vi "WirebondPatMatch.vi"(6 "Minimum Match Score":sgl, 7 "controller in":refnum<k24>, 8 "Template":path, 9 "Top or Bottom":dbl) -> (0 "error out":errorcluster, 1 "Number of Matches":i32, 3 "Match(es) Found":bool)   [LabVIEW 2011]
uses:
  <vilib>/vision/Pattern Matching.llb/IMAQ GM Match Report.ctl
  C:/Users/Admin/Desktop/Gantry Code Transfer/source/Code Transfer/Aerotech.A3200.dll
  Aerotech.A3200.dll
  Template change for pattern match.vi
  <vilib>/vision/driver/NI_Vision_Acquisition_Software.lvlib
  <vilib>/vision/NI_Vision_Development_Module.lvlib
  C:/Program Files/National Instruments/LabVIEW 2011/resource/objmgr/imaqdx.rc
panel:
  in  "Max":dbl=60.0
  in  "Min":dbl
  in  "Scale Factor":sgl=0.000429
  out "y rel move":dbl
  out "x rel move":dbl
  out "y":sgl
  out "x":sgl
  out "Image Out":T1(plugin-control)
  out "Calibrated Matches":T2[](array[typedef]) {"Correlation Score" format="%.2f"; "Target Template Curve Score" format="%.2f"; "Template Target Curve Score" format="%.2f"; "Bounding Box"."y" format="%.2f"; "Bounding Box"."x" format="%.2f"; "Position"."y" format="%.2f"; "Position"."x" format="%.2f"; "Score" format="%.2f"; "Scale" format="%.2f"; "Angle" format="%.2f"; "Occlusion %" format="%.2f"}
  out "Matches":T2[](array[typedef]) {"Correlation Score" format="%.2f"; "Target Template Curve Score" format="%.2f"; "Template Target Curve Score" format="%.2f"; "Bounding Box"."y" format="%.2f"; "Bounding Box"."x" format="%.2f"; "Position"."y" format="%.2f"; "Position"."x" format="%.2f"; "Score" format="%.2f"; "Scale" format="%.2f"; "Angle" format="%.2f"; "Occlusion %" format="%.2f"}
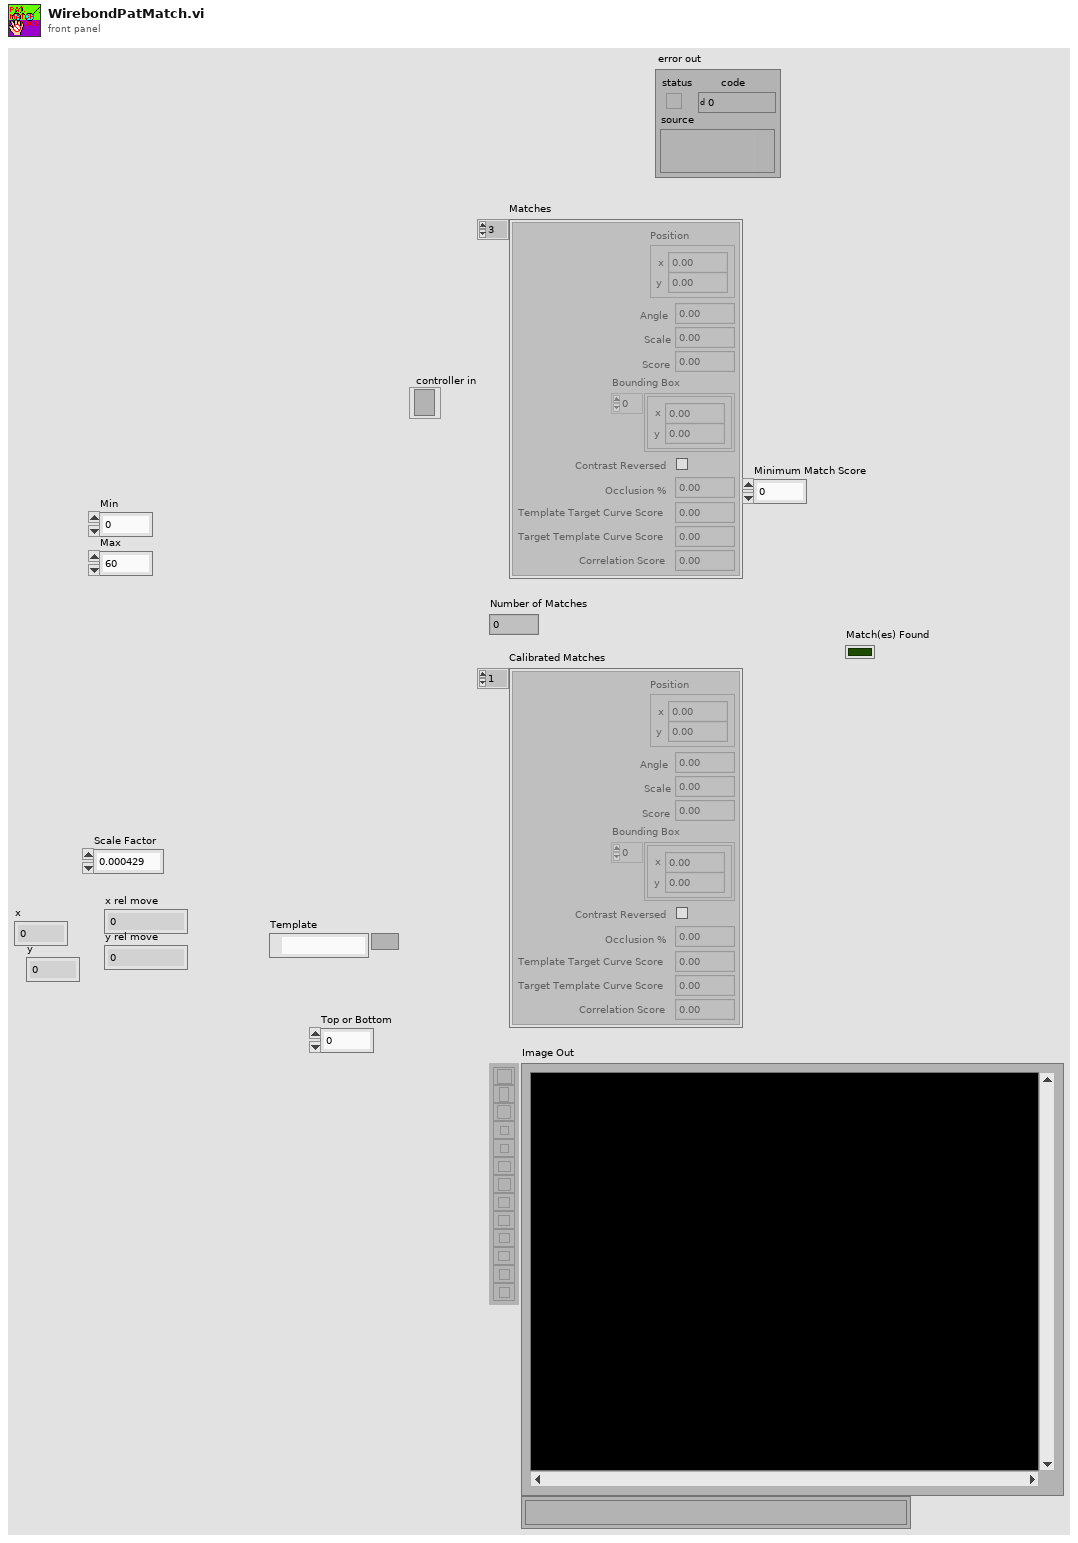
[diagram p1: front panel]
types:
  T1 = typedef "IMAQ Image.ctl" = refnum<image>
  T2 = typedef "IMAQ GM Match Report.ctl" = cluster{"Position":cluster{"x":sgl, "y":sgl}, "Angle":sgl, "Scale":sgl, "Score":sgl, "Bounding Box":cluster{"x":sgl, "y":sgl}[], "Contrast Reversed":bool, "Occlusion %":sgl, "Template Target Curve Score":sgl, "Target Template Curve Score":sgl, "Correlation Score":sgl}
  T3 = cluster{"Curve Parameters":cluster{"Extraction Mode":u32, "Edge Threshold":i32, "Edge Filter Size":u32, "Min Length":i32, "Row Search Step Size":i32, "Col Search Step Size":i32, "Max Endpoint Gap":i32, "Closed":bool, "Subpixel":bool}, "Match Mode":cluster{"Rotation":bool, "Scale":bool, "Occlusion":bool, "Reserved":bool, "Reserved":bool, "Reserved":bool}, "Range Settings":cluster{"Match Constraints":u32, "Min":dbl, "Max":dbl}[], "Number of Matches Requested":i32, "Minimum Match Score":sgl, "Subpixel Accuracy":bool}
  T4 = cluster{"Global Rectangle":i32[], "Contours":cluster{"ID":enum32{"External", "Internal"}, "Type":u32, "Coordinates":i32[]}[]}
  T5 = typedef "IMAQdx.ctl" = refnum<k21>
  T6 = cluster{"Extraction Mode":u32, "Edge Threshold":i32, "Edge Filter Size":u32, "Min Length":i32, "Row Search Step Size":i32, "Col Search Step Size":i32, "Max Endpoint Gap":i32, "Closed":bool, "Subpixel":bool}
  T7 = cluster{"Rotation":bool, "Scale":bool, "Occlusion":bool, "Reserved":bool, "Reserved":bool, "Reserved":bool}
  T8 = cluster{"Match Constraints":u32, "Min":dbl, "Max":dbl}[]
  T9 = cluster{"Match Constraints":u32, "Min":dbl, "Max":dbl}
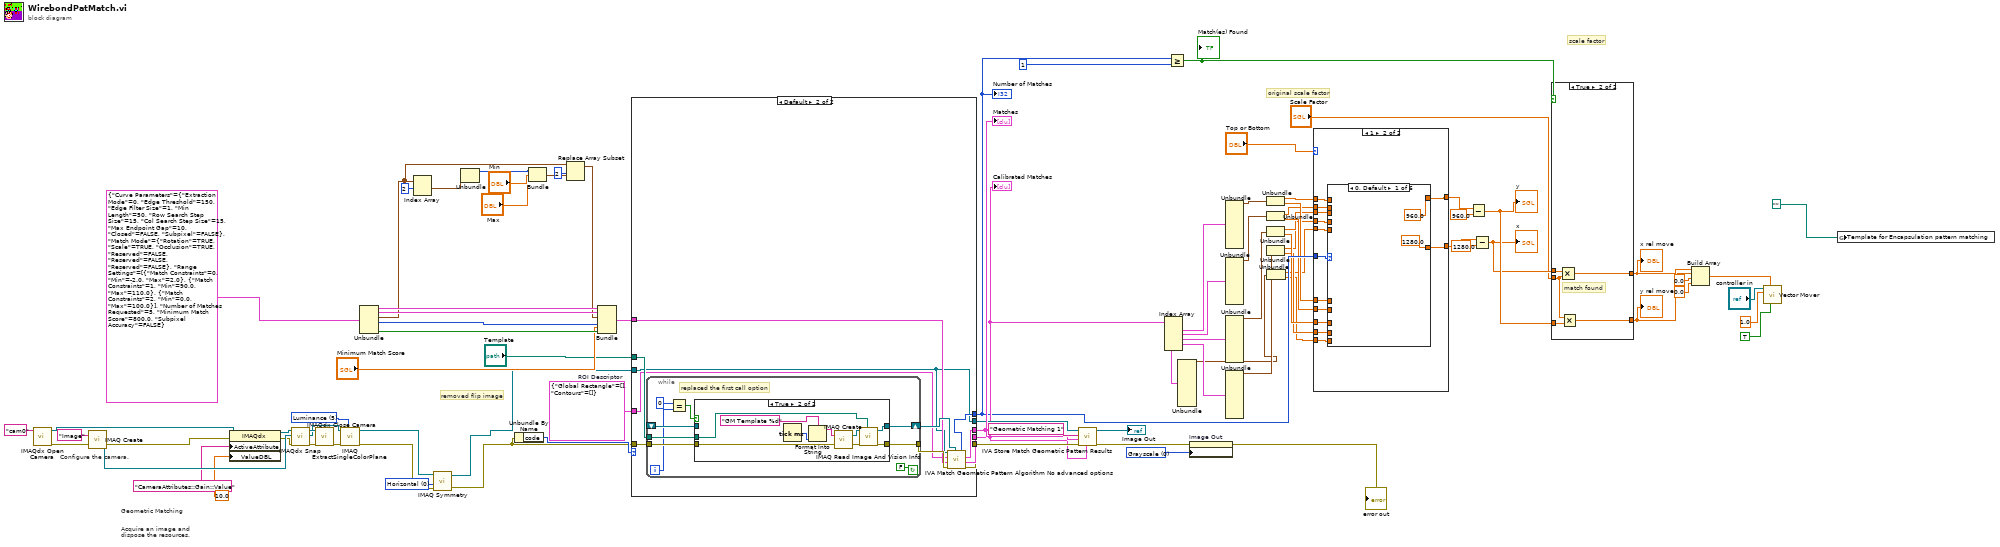
[diagram p0: block diagram]
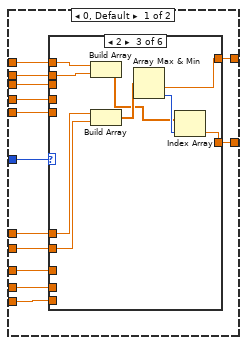
[diagram p2: hidden frame]
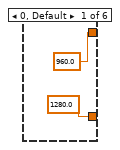
[diagram p3: hidden frame]
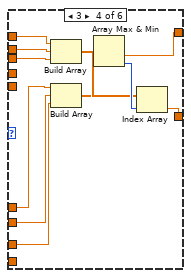
[diagram p5: hidden frame]
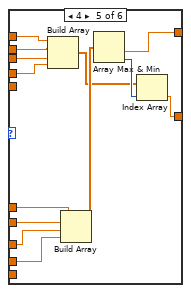
[diagram p6: hidden frame]
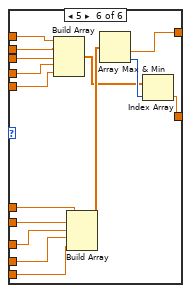
[diagram p7: hidden frame]
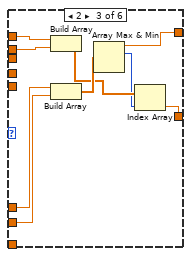
[diagram p9: hidden frame]
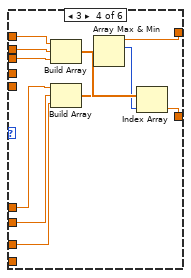
[diagram p10: hidden frame]
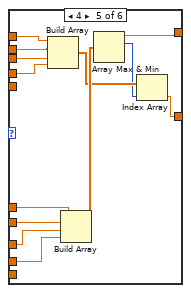
[diagram p11: hidden frame]
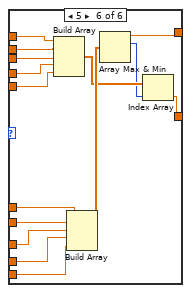
[diagram p12: hidden frame]
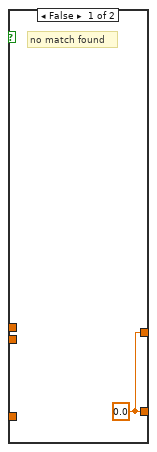
[diagram p13: hidden frame]
diagram:
  w5 = u32 0 items=["Horizontal", "Vertical", "Central", "1st Diagonal", "2nd Diagonal"] ("Type of Symmetry")
  w71 = u32 0 items=["Grayscale", "Binary", "Gradient", "Rainbow", "Temperature", "User Defined"] ("Palette")
  w79 = T4 {"Global Rectangle"=[], "Contours"=[]}  # ROI Descriptor
  w81 = 5 items=["Red", "Green", "Blue", "Hue", "Saturation", "Luminance", "Value", "Intensity"] ("Color Plane")
  # "removed flip image"
  # "original scale factor"
  # "scale factor"
  # "Geometric Matching"
  # "Acquire an image and\ndispose the resources."
  # "Configure the camera."
  n1 = call <vilib>:"IMAQdx Open Camera.vi"("Session In"="cam0" ("Interface Name")) -> ("error out"=w85:errorcluster, "Session Out"=w11:T5)  [unwired: 9 in]
  n2 = call "IMAQ Create"("Image Name"="Image", "error in (no error)"=w85) -> ("New Image"=w12:T1, "error out"=w6:errorcluster)  [unwired: 3 in]
  n3 = property class="IMAQdx"(reference=w11, error in=w6, "ActiveAttribute"="CameraAttributes::Gain::Value", "ValueDBL"=10.0) -> (reference out=w8:T5, error out=w7:errorcluster)
  n4 = call <vilib>:"IMAQdx Snap.vi"("error in"=w7, "Image In"=w12, "Session In"=w8) -> ("error out"=w83:errorcluster, "Image Out"=w80:T1, "Session Out"=w84:T5)  [unwired: 6 in]
  n5 = call <vilib>:"IMAQdx Close Camera.vi"("error in"=w83, "Session In"=w84) -> ("error out"=w82:errorcluster)  [unwired: 9 in]
  n6 = call "IMAQ ExtractSingleColorPlane"("Color Plane"=w81, "error in (no error)"=w82, "Image Src"=w80) -> ("error out"=w3:errorcluster, "Image Dst Out"=w4:T1)  [unwired: 7 in]
  n7 = Unbundle(T3 {"Curve Parameters"={"Extraction Mode"=0, "Edge Threshold"=150, "Edge Filter Size"=1, "Min Length"=50, "Row Search Step Size"=15, "Col Search Step Size"=15, "Max Endpoint Gap"=10, "Closed"=FALSE, "Subpixel"=FALSE}, "Match Mode"={"Rotation"=TRUE, "Scale"=TRUE, "Occlusion"=TRUE, "Reserved"=FALSE, "Reserved"=FALSE, "Reserved"=FALSE}, "Range Settings"=[{"Match Constraints"=0, "Min"=-2.0, "Max"=2.0}, {"Match Constraints"=1, "Min"=90.0, "Max"=110.0}, {"Match Constraints"=2, "Min"=0.0, "Max"=100.0}], "Number of Matches Requested"=5, "Minimum Match Score"=800.0, "Subpixel Accuracy"=FALSE} ("Settings (Geometric Matching 1)")) -> ("Curve Parameters"=w45:T6, "Match Mode"=w41:T7, "Range Settings"=w35:T8, "Number of Matches Requested"=w13:i32, "Subpixel Accuracy"=w44:bool)  [unwired: 1 out]
  n8 = Index Array(array=w35, index #1=2 ("index")) -> (element #1=w39:T9)  [unwired: 1 in, 1 out]
  n9 = call "IMAQ Symmetry"("error in (no error)"=w3, "Type of Symmetry"=w5, "Image Src"=w4) -> ("error out"=w2:errorcluster, "Image Dst Out"=w1:T1)  [unwired: 2 in]
  n10 = Unbundle(w39) -> ("Match Constraints"=w38:u32)  [unwired: 2 out]
  n11 = Unbundle By Name(w2) -> ("code"=w74:i32)
  n12 = Bundle("Match Constraints"=w38, "Min"="Min", "Max"="Max") -> (w34:T9)  [unwired: 1 in]
  n13 = Replace Array Subset(array=w35, new element=w34, index=2) -> (w32:T8)
  n14 = Bundle("Curve Parameters"=w45, "Match Mode"=w41, "Range Settings"=w32, "Number of Matches Requested"=w13, "Minimum Match Score"="Minimum Match Score", "Subpixel Accuracy"=w44) -> (w43:T3)  [unwired: 1 in]
  n15 = case shown="Default" w74 {
    tunnel: "Template" -> [_ w99]
    tunnel: w2 -> [_ w98]
    tunnel: w79 -> [_ w93]
    tunnel: w1 -> [w88 w92]
    tunnel: [_ w89] -> w78
    tunnel: [_ w91] -> w75
    tunnel: [_ w90] -> w65
    tunnel: [_ w97] -> w31
    tunnel: [w88 w92] -> w73
    tunnel: w43 -> [_ w94]
    frame -1074396199, -1074396198 {
      # "Discard Coordinate System Error"
    }
    frame Default {
      n16 = while {
        shift-right: [w108] -> w96
        shift-left: _ -> [w107]
        tunnel: [w105] -> w95
        tunnel: w98 -> [w104]
        tunnel: w99 -> [w103]
        i -> [w102]
        stop <- FALSE continue-if-true
        # "replaced the first call option"
        n17 = Equal?(x=0, y=w102) -> (x = y?=w100:bool)
        n18 = case shown="True" w100 {
          tunnel: [w110 w116] -> w108
          tunnel: w107 -> [w110 _]
          tunnel: [w109 w113] -> w105
          tunnel: w104 -> [w109 w112]
          tunnel: w103 -> [_ w111]
          frame False {
          }
          frame True {
            n19 = Tick Count (ms)() -> (millisecond timer value=w119:u32)
            n20 = Format Into String(format string="GM Template %d" ("Image Name"), w119) -> (resulting string=w118:string)  [unwired: 2 in, 1 out]
            n21 = call "IMAQ Create"("Image Name"=w118, "error in (no error)"=w112) -> ("New Image"=w115:T1, "error out"=w114:errorcluster)  [unwired: 3 in]
            n22 = call "IMAQ Read Image And Vision Info"("File Path"=w111, "error in (no error)"=w114, "Image"=w115) -> ("error out"=w113:errorcluster, "Image Out"=w116:T1)  [unwired: 6 in, 1 out]
          }
        }
      }
      n23 = call "IVA Match Geometric Pattern Algorithm No advanced options.vi"("Template"=w96, "error in (no error)"=w95, "Settings"=w94, "ROI Descriptor"=w93, "Image"=w92) -> ("error out"=w89:errorcluster, "Calibrated Matches"=w90:T2[], "Matches"=w91:T2[], "Number of Matches"=w97:i32)  [unwired: 3 in]
    }
  }
  "Matches" <- w75
  "Number of Matches" <- w31
  "Calibrated Matches" <- w65
  n24 = call <vilib>:"IVA Store Match Geometric Pattern Results.vi"("Calibrated Matches"=w65, "error in (no error)"=w78, "Matches"=w75, "Step Name"="Geometric Matching 1", "Image in"=w73) -> ("error out"=w77:errorcluster, "Image dup"=→"Image Out":T1)  [unwired: 5 in]
  "error out" <- w77
  n25 = Index Array(array=w65) -> (element #1=w64:T2, element #2=w63:T2, element #3=w62:T2, element #4=w61:T2, element #5=w20:T2)  [unwired: 5 in]
  n26 = Greater Or Equal?(x=w31, y=1 ("x")) -> (x >= y?=w50:bool)
  "Match(es) Found" <- w50
  n27 = Unbundle(w20) -> ("Position"=w19:cluster{"x":sgl, "y":sgl})  [unwired: 9 out]
  n28 = property on="Image Out" class="ImageControl"(error in=w77, "Palette:Palette Type"=w71) -> ()  [unwired: 1 in, 2 out]
  n29 = Unbundle(w64) -> ("Position"=w57:cluster{"x":sgl, "y":sgl})  [unwired: 9 out]
  n30 = Unbundle(w63) -> ("Position"=w58:cluster{"x":sgl, "y":sgl})  [unwired: 9 out]
  n31 = Unbundle(w62) -> ("Position"=w59:cluster{"x":sgl, "y":sgl})  [unwired: 9 out]
  n32 = Unbundle(w61) -> ("Position"=w60:cluster{"x":sgl, "y":sgl})  [unwired: 9 out]
  n33 = Unbundle(w57) -> ("x"=w30:sgl, "y"=w29:sgl)
  n34 = Unbundle(w58) -> ("x"=w28:sgl, "y"=w27:sgl)
  n35 = Unbundle(w59) -> ("x"=w25:sgl, "y"=w24:sgl)
  n36 = Unbundle(w60) -> ("x"=w21:sgl, "y"=w23:sgl)
  n37 = Unbundle(w19) -> ("x"=w18:sgl, "y"=w17:sgl)
  n38 = case shown="1" "Top or Bottom" {
    tunnel: w31 -> [w132 w185]
    tunnel: w30 -> [w131 w197]
    tunnel: w29 -> [w130 w192]
    tunnel: w28 -> [w129 w196]
    tunnel: w27 -> [w128 w191]
    tunnel: [w127 w187] -> w26
    tunnel: w25 -> [w126 w195]
    tunnel: w24 -> [w125 w190]
    tunnel: w23 -> [w124 w189]
    tunnel: [w123 w186] -> w22
    tunnel: w21 -> [w122 w194]
    tunnel: w18 -> [w121 w193]
    tunnel: w17 -> [w120 w188]
    frame 0, Default {
      n39 = case shown="2" w132 {
        tunnel: w131 -> [_ w135 w145 w153 w166 w181]
        tunnel: w130 -> [_ w136 w143 w150 w162 w177]
        tunnel: [sgl 960.0 ("y") w136 w140 w155 w168 w183] -> w127
        tunnel: w129 -> [_ _ w144 w152 w165 w180]
        tunnel: w128 -> [_ _ w142 w149 w161 w176]
        tunnel: w126 -> [_ _ _ w151 w164 w179]
        tunnel: w125 -> [_ _ _ w148 w160 w175]
        tunnel: w124 -> [_ _ _ _ w159 w174]
        tunnel: [sgl 1280.0 ("x") w135 w137 w154 w167 w182] -> w123
        tunnel: w122 -> [_ _ _ _ w163 w178]
        tunnel: w121 -> [_ _ _ _ _ w171]
        tunnel: w120 -> [_ _ _ _ _ w170]
        frame 0, Default {
        }
        frame 1 {
        }
        frame 2 {
          n40 = Build Array(w145, w144) -> (w138:sgl[])
          n41 = Build Array(w143, w142) -> (w139:sgl[])
          n42 = Array Max & Min(array=w139) -> (min value=w140:sgl, min index (indices)=w141:i32)  [unwired: 2 out]
          n43 = Index Array(array=w138, index=w141) -> (element=w137:sgl)
        }
        frame 3 {
          n44 = Build Array(w153, w152, w151) -> (w147:sgl[])
          n45 = Build Array(w150, w149, w148) -> (w146:sgl[])
          n46 = Array Max & Min(array=w146) -> (min value=w155:sgl, min index (indices)=w156:i32)  [unwired: 2 out]
          n47 = Index Array(array=w147, index=w156) -> (element=w154:sgl)
        }
        frame 4 {
          n48 = Build Array(w166, w165, w164, w163) -> (w157:sgl[])
          n49 = Build Array(w162, w161, w160, w159) -> (w158:sgl[])
          n50 = Array Max & Min(array=w158) -> (min value=w168:sgl, min index (indices)=w169:i32)  [unwired: 2 out]
          n51 = Index Array(array=w157, index=w169) -> (element=w167:sgl)
        }
        frame 5 {
          n52 = Build Array(w181, w180, w179, w178, w171) -> (w172:sgl[])
          n53 = Build Array(w177, w176, w175, w174, w170) -> (w173:sgl[])
          n54 = Array Max & Min(array=w173) -> (min value=w183:sgl, min index (indices)=w184:i32)  [unwired: 2 out]
          n55 = Index Array(array=w172, index=w184) -> (element=w182:sgl)
        }
      }
    }
    frame 1 {
      n56 = case shown="0, Default" w185 {
        tunnel: w197 -> [_ w200 w210 w220 w233 w248]
        tunnel: w192 -> [_ w201 w208 w217 w229 w244]
        tunnel: [sgl 960.0 ("y") w201 w203 w212 w223 w236] -> w187
        tunnel: w196 -> [_ _ w209 w219 w232 w247]
        tunnel: w191 -> [_ _ w207 w216 w228 w243]
        tunnel: w195 -> [_ _ _ w218 w231 w246]
        tunnel: w190 -> [_ _ _ w215 w227 w242]
        tunnel: w189 -> [_ _ _ _ w226 w241]
        tunnel: [sgl 1280.0 ("x") w200 w204 w221 w234 w249] -> w186
        tunnel: w194 -> [_ _ _ _ w230 w245]
        tunnel: w193 -> [_ _ _ _ _ w238]
        tunnel: w188 -> [_ _ _ _ _ w237]
        frame 0, Default {
        }
        frame 1 {
        }
        frame 2 {
          n57 = Build Array(w210, w209) -> (w205:sgl[])
          n58 = Build Array(w208, w207) -> (w206:sgl[])
          n59 = Array Max & Min(array=w206) -> (max value=w203:sgl, max index (indices)=w202:i32)  [unwired: 2 out]
          n60 = Index Array(array=w205, index=w202) -> (element=w204:sgl)
        }
        frame 3 {
          n61 = Build Array(w220, w219, w218) -> (w214:sgl[])
          n62 = Build Array(w217, w216, w215) -> (w213:sgl[])
          n63 = Array Max & Min(array=w213) -> (max value=w212:sgl, max index (indices)=w211:i32)  [unwired: 2 out]
          n64 = Index Array(array=w214, index=w211) -> (element=w221:sgl)
        }
        frame 4 {
          n65 = Build Array(w233, w232, w231, w230) -> (w224:sgl[])
          n66 = Build Array(w229, w228, w227, w226) -> (w225:sgl[])
          n67 = Array Max & Min(array=w225) -> (max value=w223:sgl, max index (indices)=w222:i32)  [unwired: 2 out]
          n68 = Index Array(array=w224, index=w222) -> (element=w234:sgl)
        }
        frame 5 {
          n69 = Build Array(w248, w247, w246, w245, w238) -> (w239:sgl[])
          n70 = Build Array(w244, w243, w242, w241, w237) -> (w240:sgl[])
          n71 = Array Max & Min(array=w240) -> (max value=w236:sgl, max index (indices)=w235:i32)  [unwired: 2 out]
          n72 = Index Array(array=w239, index=w235) -> (element=w249:sgl)
        }
      }
    }
  }
  n73 = Subtract(x=w26, y=sgl 960.0) -> (x-y=w68:sgl)
  "y" <- w68
  n74 = Subtract(x=w22, y=sgl 1280.0) -> (x-y=w67:sgl)
  "x" <- w67
  n75 = case shown="True" w50 {
    tunnel: w68 -> [_ w255]
    tunnel: w67 -> [_ w254]
    tunnel: [w250 w253] -> w48
    tunnel: [w250 w252] -> w49
    tunnel: "Scale Factor" -> [_ w251]
    frame False {
      w250 = sgl 0.0
      # "no match found"
    }
    frame True {
      # "match found"
      n76 = Multiply(x=w254, y=w251) -> (x*y=w253:sgl)
      n77 = Multiply(x=w251, y=w255) -> (x*y=w252:sgl)
    }
  }
  "x rel move" <- w48
  "y rel move" <- w49
  n78 = Build Array(w49, w48, 0.0 ("element"), 0.0 ("element")) -> (w51:dbl[])
  n79 = call "Vector Mover.vi"("Absolute/Relative (F/T)"=TRUE, "Movement Vector"=w51, "Vector Speed"=1.0, "controller in"="controller in") -> ()  [unwired: 2 in, 4 out]
  n80 = global write "Template change for pattern match.vi" "Template for Encapsulation pattern matching"(path "") -> ()
